vi "SSC DAQmx Read (Analog 1D Wfm).vi"(0 "DAQmx SSC in":T1[](array[typedef]), 5 "Samples to read":i32=-1, 11 "error in":errorcluster) -> (4 "DAQmx SSC out":T1[](array[typedef]), 6 "Per-Task Waveforms out":waveform(dbl)[][](array[waveform]), 15 "error out":errorcluster)   [LabVIEW 2020]
doc: "Reads one or more waveforms from a task that contains one or more analog input channels. The data will be ordered based on the SSC order."
uses:
  Pin Map/SSC DAQmx.ctl
  <vilib>/DAQmx/read.llb/DAQmx Read (Analog 1D Wfm NChan NSamp).vi
  <vilib>/DAQmx/miscellaneous.llb/DAQmx Fill In Error Info.vi
  <resource>/objmgr/daqmx.rc
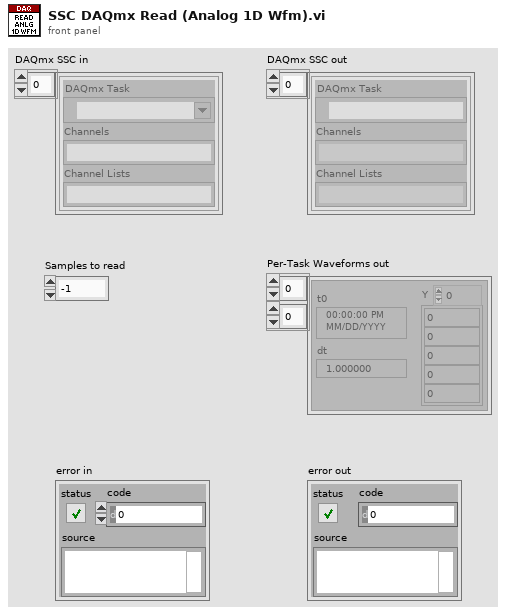
[diagram p1: front panel]
types:
  T1 = typedef "SSC DAQmx.ctl" = cluster{"DAQmx Task ":refnum<k21>, "Channels":string, "Channel Lists":string}
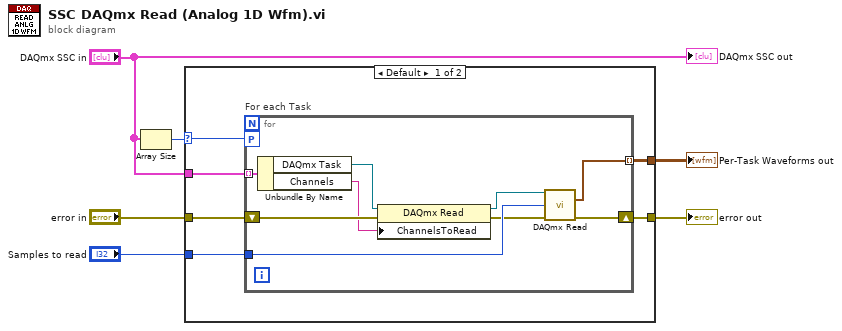
[diagram p0: block diagram]
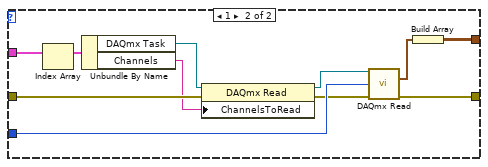
[diagram p2: hidden frame]
diagram:
  n1 = Array Size(array="DAQmx SSC in") -> (size(s)=w4:i32)
  n2 = case shown="Default" w4 {
    selector: w4 -> [w7 _]
    tunnel: "error in" -> [w12 w32]
    tunnel: "Samples to read" -> [w11 w31]
    tunnel: [w10 w22] -> w5
    tunnel: "DAQmx SSC in" -> [w8 w29]
    tunnel: [w9 w28] -> w3
    frame Default {
      n3 = for "For each Task" {
        tunnel: [w21] -> w10 mode=indexing
        shift-right: [w19] -> w9
        shift-left: w12 -> [w20]
        workers-P: w7 -> [_]
        tunnel: w11 -> [w18]
        tunnel: w8 -> [w17] mode=indexing
        n4 = Unbundle By Name(w17) -> ("DAQmx Task"=w14:refnum<k21>, "Channels"=w15:string)
        n5 = property class="DAQmx Read"(reference=w14, error in=w20, "ChannelsToRead"=w15) -> (reference out=w13:refnum<k21>, error out=w16:errorcluster)
        n6 = call-poly <vilib>:"DAQmx Read.vi"("task/channels in"=w13, "number of samples per channel"=w18, "error in"=w16) -> ("data"=w21:waveform(dbl)[], "error out"=w19:errorcluster)  [unwired: 10 in, 1 out]
      }
    }
    frame 1 {
      n7 = Index Array(array=w29) -> (element=w23:T1)  [unwired: 1 in]
      n8 = Unbundle By Name(w23) -> ("DAQmx Task"=w25:refnum<k21>, "Channels"=w26:string)
      n9 = property class="DAQmx Read"(reference=w25, error in=w32, "ChannelsToRead"=w26) -> (reference out=w24:refnum<k21>, error out=w27:errorcluster)
      n10 = call-poly <vilib>:"DAQmx Read.vi"("task/channels in"=w24, "number of samples per channel"=w31, "error in"=w27) -> ("data"=w30:waveform(dbl)[], "error out"=w28:errorcluster)  [unwired: 10 in, 1 out]
      n11 = Build Array(w30) -> (w22:waveform(dbl)[][])
    }
  }
  "Per-Task Waveforms out" <- w5
  "error out" <- w3
  "DAQmx SSC out" <- "DAQmx SSC in"
